vi "USRP Packet Receiver_Queue.vi"() -> ()   [LabVIEW 2013]
uses:
  <vilib>/addons/Modulation/niDMT.lvlib
panel:
  in  "16-PSK System Parameters":T1={"Samples per Symbol"=8, "symbol map"=[], "Differential PSK"=enum."disable", "PSK type"=0} {"PSK type" items=["normal", "shifted", "offset"]; "symbol map" format="%.3f"}
  in  "8-PSK System Parameters":T1={"Samples per Symbol"=8, "symbol map"=[], "Differential PSK"=enum."disable", "PSK type"=0} {"PSK type" items=["normal", "shifted", "offset"]; "symbol map" format="%.3f"}
  in  "QPSK System Parameters":T1={"Samples per Symbol"=8, "symbol map"=[], "Differential PSK"=enum."disable", "PSK type"=0} {"PSK type" items=["normal", "shifted", "offset"]; "symbol map" format="%.3f"}
  in  "BPSK System Parameters":T1={"Samples per Symbol"=8, "symbol map"=[], "Differential PSK"=enum."disable", "PSK type"=0} {"PSK type" items=["normal", "shifted", "offset"]; "symbol map" format="%.3f"}
  out "Sync Found":bool
  out "Recovered Message":string
  out "Received Signal (Raw)":dbl[](graph)
  out "Constellation Graph":T2(graph)
  in  "filter parameters":T3={"Alpha"=0.5, "Filter Length"=6, "TX Filter"=enum."Root Raised Cos"} caption="Matching Filter Parameters" {"Alpha" format="%.2f"}
  in  "Modulation type":string(combo)="QPSK"
  in  "Rx IQ Sampling\nRate [s/sec]":dbl=400000.0 format="%#.6p"
  out "Symbol Rate [symbols/sec]":dbl=25000.0 format="%#.6p"
  out "Correct Packets Rx":i16
  in  "Continuous Acquire?":bool
  out "Singal & Noise Power":cluster{"signal_power":dbl, "noise_power":dbl}={"signal_power"=1.4546950663593878e-09, "noise_power"=2.571229598792933e-12}
  out "Cumulative Packets Recovered":i16(graph)
  out "Signal and Noise Power Tracking":cluster{"total_power":dbl, "noise_power":dbl}(graph)={"total_power"=1.4546950663593878e-09, "noise_power"=2.571229598792933e-12}
  in  "PN Sequence Order for Sync":i32=31
  in  "Packet Parameters":T4={"Guard Bits "=30, "Sync Bits"=20, "Message Bits"=128, "Number of Packets \nto Expect"=46}
  in  "synchronization parameters":T5={"expected sync location (symbols)"=-1, "sync sequence"=[], "sync location uncertainty (symbols)"=0, "sync indent (symbols)"=0} {"sync sequence" format="%.2f"}
  in  "stop":bool
  # "Guard\nBand"
  # "Sync\nSeq"
  # "Packet\nNumber"
  # "Pad\nData"
  # "Data"
  # "Packet Receiver"
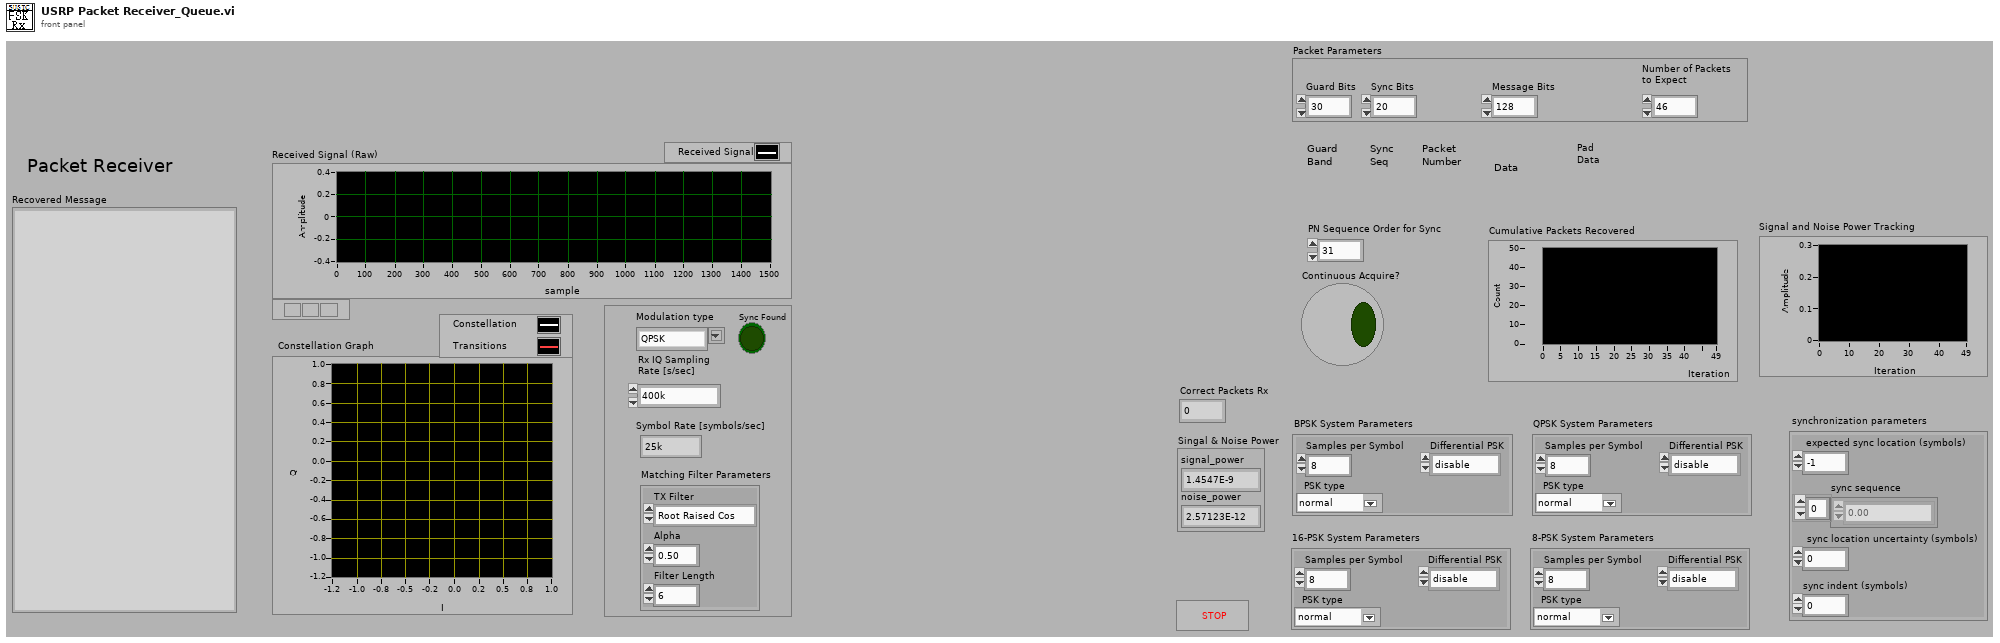
[diagram p1: front panel]
types:
  T1 = cluster{"Samples per Symbol":i32, "symbol map":cdb[], "Differential PSK":enum16{"disable", "enable"}, "PSK type":u16}
  T2 = cluster{"Decimated Array":dbl[], "Decimated Array":dbl[]}[]
  T3 = cluster{"Alpha":dbl, "Filter Length":i32, "TX Filter":enum16{"none", "Raised Cosine", "Root Raised Cos", "Gaussian"}}
  T4 = cluster{"Guard Bits ":i32, "Sync Bits":i32, "Message Bits":i32, "Number of Packets \nto Expect":i32}
  T5 = cluster{"expected sync location (symbols)":i32, "sync sequence":cdb[], "sync location uncertainty (symbols)":i32, "sync indent (symbols)":i32}
  T6 = cluster{"Packet Array":i32[][], "IP Array of Pkt Nums Received  ":bool[]}
  T7 = cluster{"bit stream ":i8[][], "Sync Valid?":bool[], "Decoded Pkt Numbers":u32[], "Enable?":bool}
  T8 = cluster{"packet_arr":cdb[][], "Packets Valid?":bool}
  T9 = cluster{"PSK type":u16, "Samples per Symbol":i32, "Differential PSK":enum16{"disable", "enable"}, "M-PSK (4)":i32}
  T10 = cluster{"PSK system parameters":cluster{"samples per symbol (16)":i32, "symbol map":cdb[], "differential PSK":enum16{"disable", "enable"}, "PSK type":u16}, "pulse shaping filter coefficients":dbl[], "matched filter coefficients":dbl[], "synchronization parameters":cluster{"expected sync location (symbols)":i32, "sync sequence":cdb[], "sync location uncertainty (symbols)":i32, "sync indent (symbols)":i32}, "Sync Bits":i8[]}
  T11 = typedef "niAMT.lvlib/Complex Data Waveform.ctl" = cluster{"t0":dbl, "dt":dbl, "Y":cdb[]}
  T12 = cluster{"constellation":dbl[], "oversampled data":dbl[]}[]
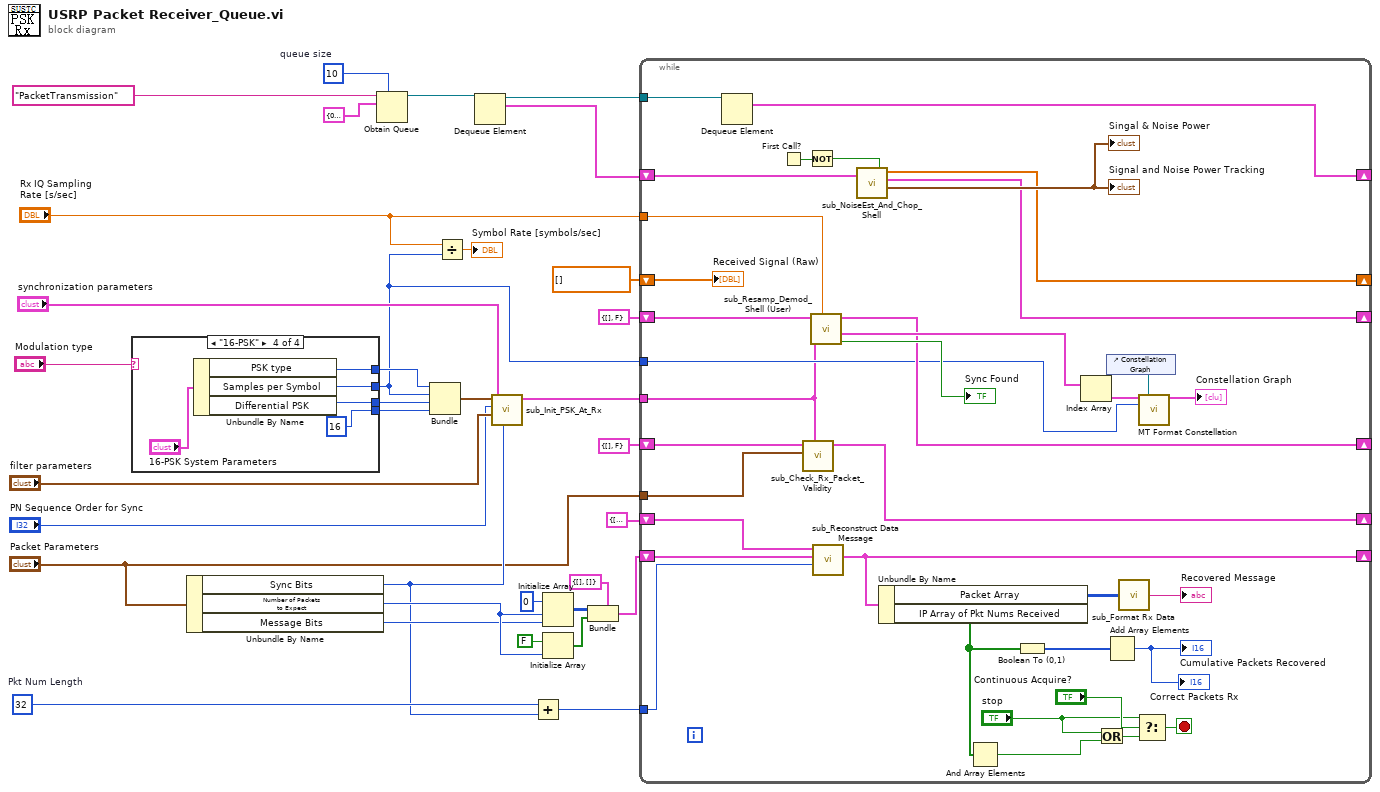
[diagram p0: block diagram]
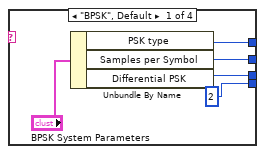
[diagram p2: hidden frame]
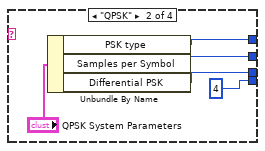
[diagram p3: hidden frame]
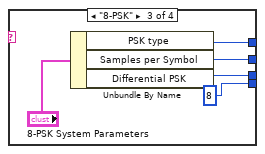
[diagram p4: hidden frame]
diagram:
  w7 = 10  # queue size
  w24 = 32  # Pkt Num Length
  n1 = case shown="\"16-PSK\"" "Modulation type" {
    tunnel: [w37 w43 w48 w54] -> w1
    tunnel: [w38 w41 w47 w53] -> w30
    tunnel: [2 ("M-PSK (4)") 4 ("M-PSK (4)") 8 ("M-PSK (4)") 16 ("M-PSK (4)")] -> w29
    tunnel: [w39 w42 w49 w52] -> w31
    frame "BPSK", Default {
      n2 = Unbundle By Name("BPSK System Parameters") -> ("PSK type"=w39:u16, "Samples per Symbol"=w37:i32, "Differential PSK"=w38:enum16{"disable", "enable"})
    }
    frame "QPSK" {
      n3 = Unbundle By Name("QPSK System Parameters") -> ("PSK type"=w42:u16, "Samples per Symbol"=w43:i32, "Differential PSK"=w41:enum16{"disable", "enable"})
    }
    frame "8-PSK" {
      n4 = Unbundle By Name("8-PSK System Parameters") -> ("PSK type"=w49:u16, "Samples per Symbol"=w48:i32, "Differential PSK"=w47:enum16{"disable", "enable"})
    }
    frame "16-PSK" {
      n5 = Unbundle By Name("16-PSK System Parameters") -> ("PSK type"=w52:u16, "Samples per Symbol"=w54:i32, "Differential PSK"=w53:enum16{"disable", "enable"})
    }
  }
  n6 = Unbundle By Name("Packet Parameters") -> ("Sync Bits"=w15:i32, "Number of Packets \nto Expect"=w23:i32, "Message Bits"=w22:i32)
  n7 = Obtain Queue(max queue size (-1, unlimited)=w7, name (unnamed)="PacketTransmission", element data type=cluster{"t0":dbl, "dt":dbl, "Y":cdb[]} {"t0"=0.0, "dt"=0.0, "Y"=[]} ("s? t:f")) -> (queue out=w9:refnum<queue>)  [unwired: 2 in, 2 out]
  n8 = Bundle("PSK type"=w31, "Samples per Symbol"=w1, "Differential PSK"=w30, "M-PSK (4)"=w29) -> (w27:T9)  [unwired: 1 in]
  n9 = Divide(x="Rx IQ Sampling\nRate [s/sec]", y=w1) -> (x/y=→"Symbol Rate [symbols/sec]":dbl)
  n10 = Dequeue Element(queue=w9) -> (queue out=w8:refnum<queue>, element=w5:cluster{"t0":dbl, "dt":dbl, "Y":cdb[]})  [unwired: 2 in, 2 out]
  n11 = call "sub_Init_PSK_At_Rx.vi"("Sync Bits"=w15, "synchronization parameters"="synchronization parameters", "filter parameters"="filter parameters", "PN sequence order (9)"="PN Sequence Order for Sync", "PSK Parameters"=w27) -> ("PSK Init Parameters"=w26:T10)  [unwired: 5 in, 1 out]
  n12 = Add(x=w24, y=w15) -> (x+y=w32:i32)
  n13 = Initialize Array(0, w23, w22) -> (w17:i32[][])
  n14 = Initialize Array(FALSE, w23) -> (w16:bool[])
  n15 = Bundle(cluster=T6 {"Packet Array"=[], "IP Array of Pkt Nums Received  "=[]} ("Packet Info"), "Packet Array"=w17, "IP Array of Pkt Nums Received"=w16) -> (w12:T6)
  n16 = while {
    tunnel: "Rx IQ Sampling\nRate [s/sec]" -> [w90]
    tunnel: "Packet Parameters" -> [w89]
    tunnel: w32 -> [w66]
    tunnel: w26 -> [w59]
    tunnel: w1 -> [w60]
    shift-right: [w64] -> _
    shift-left: w12 -> [w67]
    shift-right: [w72] -> _
    shift-left: T8 {"packet_arr"=[], "Packets Valid?"=FALSE} -> [w73]
    shift-right: [w69] -> _
    shift-left: cluster{"bit stream":i8[][], "Enable?":bool} {"bit stream"=[], "Enable?"=FALSE} ("Output Bitstream") -> [w71]
    shift-right: [w58] -> _
    shift-left: T7 {"bit stream "=[], "Sync Valid?"=[], "Decoded Pkt Numbers"=[], "Enable?"=FALSE} ("Output Bit Stream") -> [w68]
    shift-right: [w55] -> _
    shift-left: w5 -> [w70]
    shift-right: [w61] -> _
    shift-left: cdb[] [] ("Delay signal (for plotting use only)") -> [w62]
    tunnel: w8 -> [w56]
    stop <- w85 stop-if-true
    n17 = Dequeue Element(queue=w56) -> (element=w55:cluster{"t0":dbl, "dt":dbl, "Y":cdb[]})  [unwired: 2 in, 3 out]
    n18 = First Call?() -> (First Call?: T/F=w76:bool)
    n19 = call "sub_Check_Rx_Packet_Validity.vi"("PSK Init Parameters"=w59, "Packet Parameters"=w89, "Input Bit Stream"=w71) -> ("Output Bit Stream"=w58:T7)  [unwired: 7 in]
    n20 = Not(x=w76) -> (.not. x?=w75:bool)
    n21 = call "sub_Resamp_Demod_Shell (User).vi"("Rx IQ Sampling\nRate [s/sec]"=w90, "PSK Init Parameters"=w59, "Input Packets"=w73) -> ("Synch Found?"=→"Sync Found":bool, "recovered complex waveform"=w78:T11[], "Output Bitstream"=w69:cluster{"bit stream":i8[][], "Enable?":bool})  [unwired: 3 in]
    n22 = call "sub_Reconstruct Data Message.vi"("Start Loc of Data"=w66, "Packet Info"=w67, "Input Stream"=w68) -> ("Packet Info out"=w64:T6)  [unwired: 8 in]
    n23 = call "sub_NoiseEst_And_Chop_Shell.vi"("data"=w70, "Enable"=w75) -> ("Singal & Noise Power"=→"Signal and Noise Power Tracking" →"Singal & Noise Power":cluster{"signal_power":dbl, "noise_power":dbl}, "Output Packets"=w72:cluster{"Packets":cdb[][], "Enable?":bool}, "Delay signal (for plotting use only)"=w61:cdb[])  [unwired: 3 in]
    n24 = Unbundle By Name(w64) -> ("Packet Array"=w65:i32[][], "IP Array of Pkt Nums Received"=w63:bool[])
    n25 = And Array Elements(Boolean array=w63) -> (logical AND=w57:bool)
    n26 = Boolean To (0,1)(Boolean=w63) -> (0, 1=w88:i16[])
    n27 = Index Array(array=w78) -> (element=w77:T11)  [unwired: 1 in]
    n28 = Or(x="stop", y=w57) -> (x .or. y?=w86:bool)
    n29 = control-ref of="Constellation Graph"() -> (w80:refnum<vi>)
    n30 = Add Array Elements(numeric array=w88) -> (sum=→"Correct Packets Rx" →"Cumulative Packets Recovered":i16)
    n31 = call "sub_Format Rx Data.vi"("Output Packet Array"=w65) -> ("Received Message"=→"Recovered Message":string)
    n32 = Select(t="stop", s="Continuous Acquire?", f=w86) -> (s? t:f=w85:bool)
    n33 = call <vilib>:"MT Format Constellation.vi"("waveform"=w77, "constellation reference"=w80, "samples per symbol"=w60) -> ("constellation graph"=→"Constellation Graph":T12)  [unwired: 2 in, 10 out]
    "Received Signal (Raw)" <- w62
  }
